vi "烧录座位置补偿设定界面.vi"(8 "错误输入（无错误）":errorcluster, 10 "界面切换队列":refnum<queue>, 11 "VISA资源名称输入":refnum<visa-resource-name>) -> (0 "错误输出":errorcluster, 3 "VISA资源名称输出":refnum<visa-resource-name>)   [LabVIEW 2018]
panel:
  out "毫秒计时值":u32
  in  "枚举":T1(ring)
  in  "选项卡控件":enum32{"选项卡 1", "选项卡 2"}(tab)
  out "吸嘴偏移参数界面":bool
  out "写DDT32480":dbl
  out "写DDT32430":dbl
  out "写DDT32478":dbl
  out "写DDT32428":dbl
  out "写DDT32476":dbl
  out "写DDT32426":dbl
  out "写DDT32474":dbl
  out "写DDT32424":dbl
  out "写DDT32472":dbl
  out "写DDT32422":dbl
  out "写DDT32470":dbl
  out "写DDT32420":dbl
  out "写DDT32468":dbl
  out "写DDT32418":dbl
  out "写DDT32466":dbl
  out "写DDT32416":dbl
  out "写DDT32464":dbl
  out "写DDT32414":dbl
  out "写DDT32462":dbl
  out "写DDT32412":dbl
  out "写DDT32460":dbl
  out "写DDT32410":dbl
  out "写DDT32458":dbl
  out "写DDT32408":dbl
  out "写DDT32456":dbl
  out "写DDT32406":dbl
  out "写DDT32454":dbl
  out "写DDT32404":dbl
  out "写DDT32452":dbl
  out "写DDT32402":dbl
  out "写DDT32450":dbl
  out "写DDT32400":dbl
  out "DDT90356":dbl
  out "DDT90348":dbl
  out "自动界面":bool
  out "手动界面":bool
  out "参数界面":bool
  out "IO界面":bool
  out "产品界面":bool
  out "字符串":string
  out "DDT90352":dbl
  out "DDT90360":dbl
  out "通讯周期":dbl
  out "DT1184":T2(ring)
  out "写R0+读R1+手动启动":bool
  out "写R4+读R4+手动停止":bool
  out "写R8+读R9+机器复位":bool
  # "X"
  # "Z1"
  # "Z2"
  # "Y"
  # "Y轴"
  # "Y轴"
  # "X轴"
  # "X轴"
  # "烧录座补偿"
  # "09"
  # "01"
  # "只有光标\n对位模式下\n补偿才有用"
  # "10"
  # "02"
  # "11"
  # "03"
  # "要多走一点\n就设正值\n要少走一点\n就设负值\n比如要多走1MM\n就设1.00\n如果想要少走1MM\n就设-1.00"
  # "12"
  # "04"
  # "13"
  # "05"
  # "14"
  # "06"
  # "15"
  # "07"
  # "16"
  # "08"
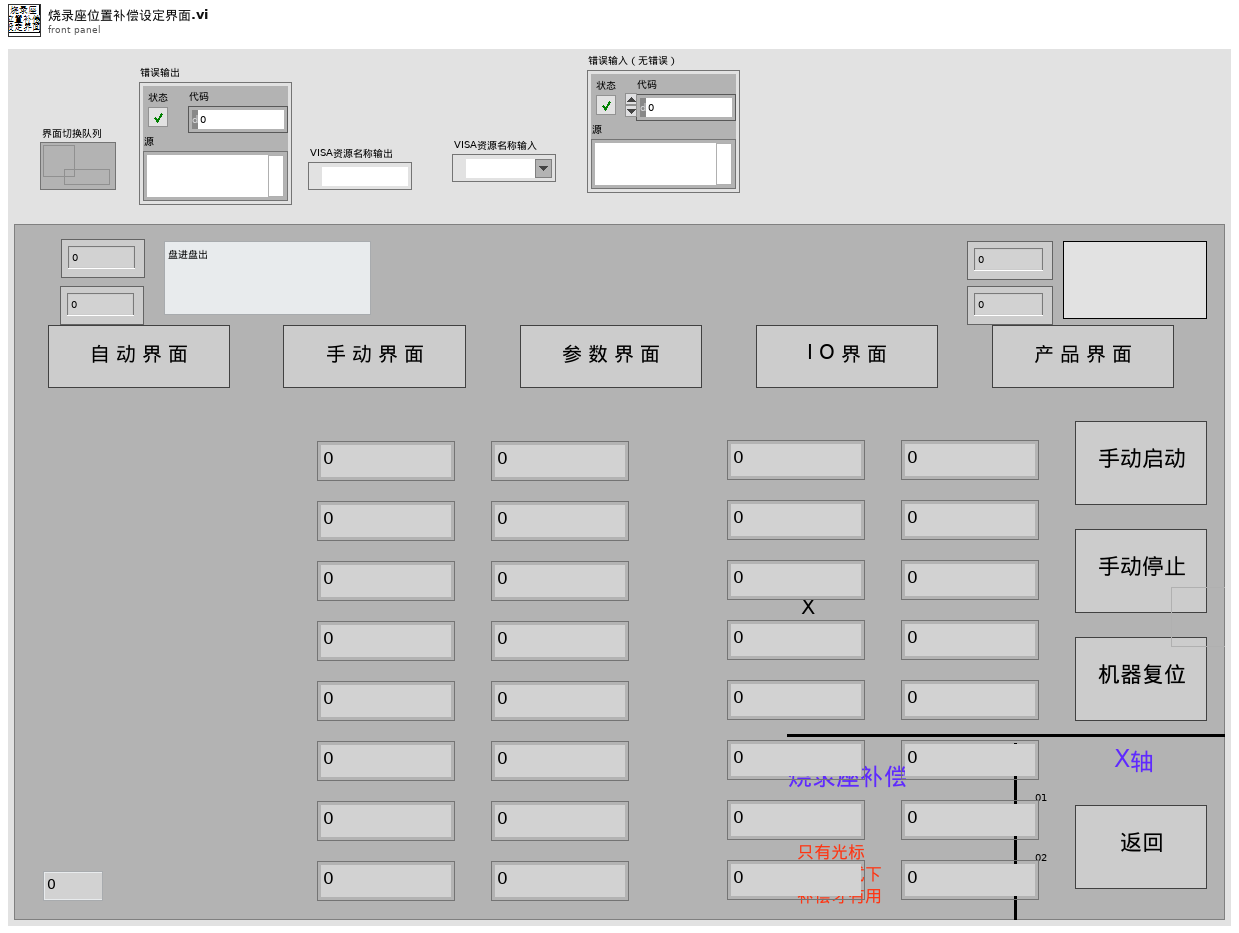
[diagram p1: front panel]
types:
  T1 = enum16{"读初始化", "读R9+8", "读R1+8", "读DDT32480", "读DDT32470+5", "读DDT32460+5", "读DDT32450+5", "读DDT32430", "读DDT32420+5", "读DDT32410+5", "读DDT32400+5", "读DDT90356", "读DT1184", "读DDT90348", ""}
  T2 = enum16{"盘进盘出", "卷进卷出", "盘进卷出", "管进盘出", "管进卷出", "卷进盘出", ""}
  T3 = enum8{"Enabled", "Disabled", "Disabled and Grayed Out"}
  T4 = typedef "数据簇.ctl" = cluster{"字符串":string, "数值":i32, "布尔":bool}
  T5 = typedef "lveventtype.ctl" = enum32{"Null", "Timeout", "Annotation Menu Selection", "Annotation Menu Selection?", "App Instance Close", "App Instance Close?", "Autoscale Range Change", "Bookmark Info Change", "Cell Edit", "Cell Edit?", "Cursor Grab", "Cursor Grab?", "Cursor Menu Selection", "Cursor Menu Selection?", "Cursor Move", "Cursor Release", "Data Change", "Direction Change", "Display State Change", "Drag Ended", "Drag Enter", "Drag Leave", "Drag Over", "Drag Source Update", "Drag Starting", "Drag Starting?", "Drop", "Exec State Change", "Key Down", "Key Down?", "Key Repeat", "Key Repeat?", "Key Up", "Listbox Double Click", "Menu Activation?", "Menu Selection (App)", "Menu Selection? (App)", "Menu Selection (User)", "Mouse Down", "Mouse Down?", "Mouse Enter", "Mouse Leave", "Mouse Move", "Mouse Up", "Mouse Wheel", "NI Security User Change (App)", "Pane Size", "Panel Close", "Panel Close?", "Panel Resize", "Plot Attribute Change", "Scale Range Change", "Shortcut Menu Activation?", "Shortcut Menu Selection (App)", "Shortcut Menu Selection? (App)", "Shortcut Menu Selection (User)", "Tree Double Click", "Tree Drag", "Tree Drag?", "Tree Drop", "Tree Drop?", "Tree Item Close", "Tree Item Close?", "Tree Item Open", "Tree Item Open?", "User Event", "Value Change"}
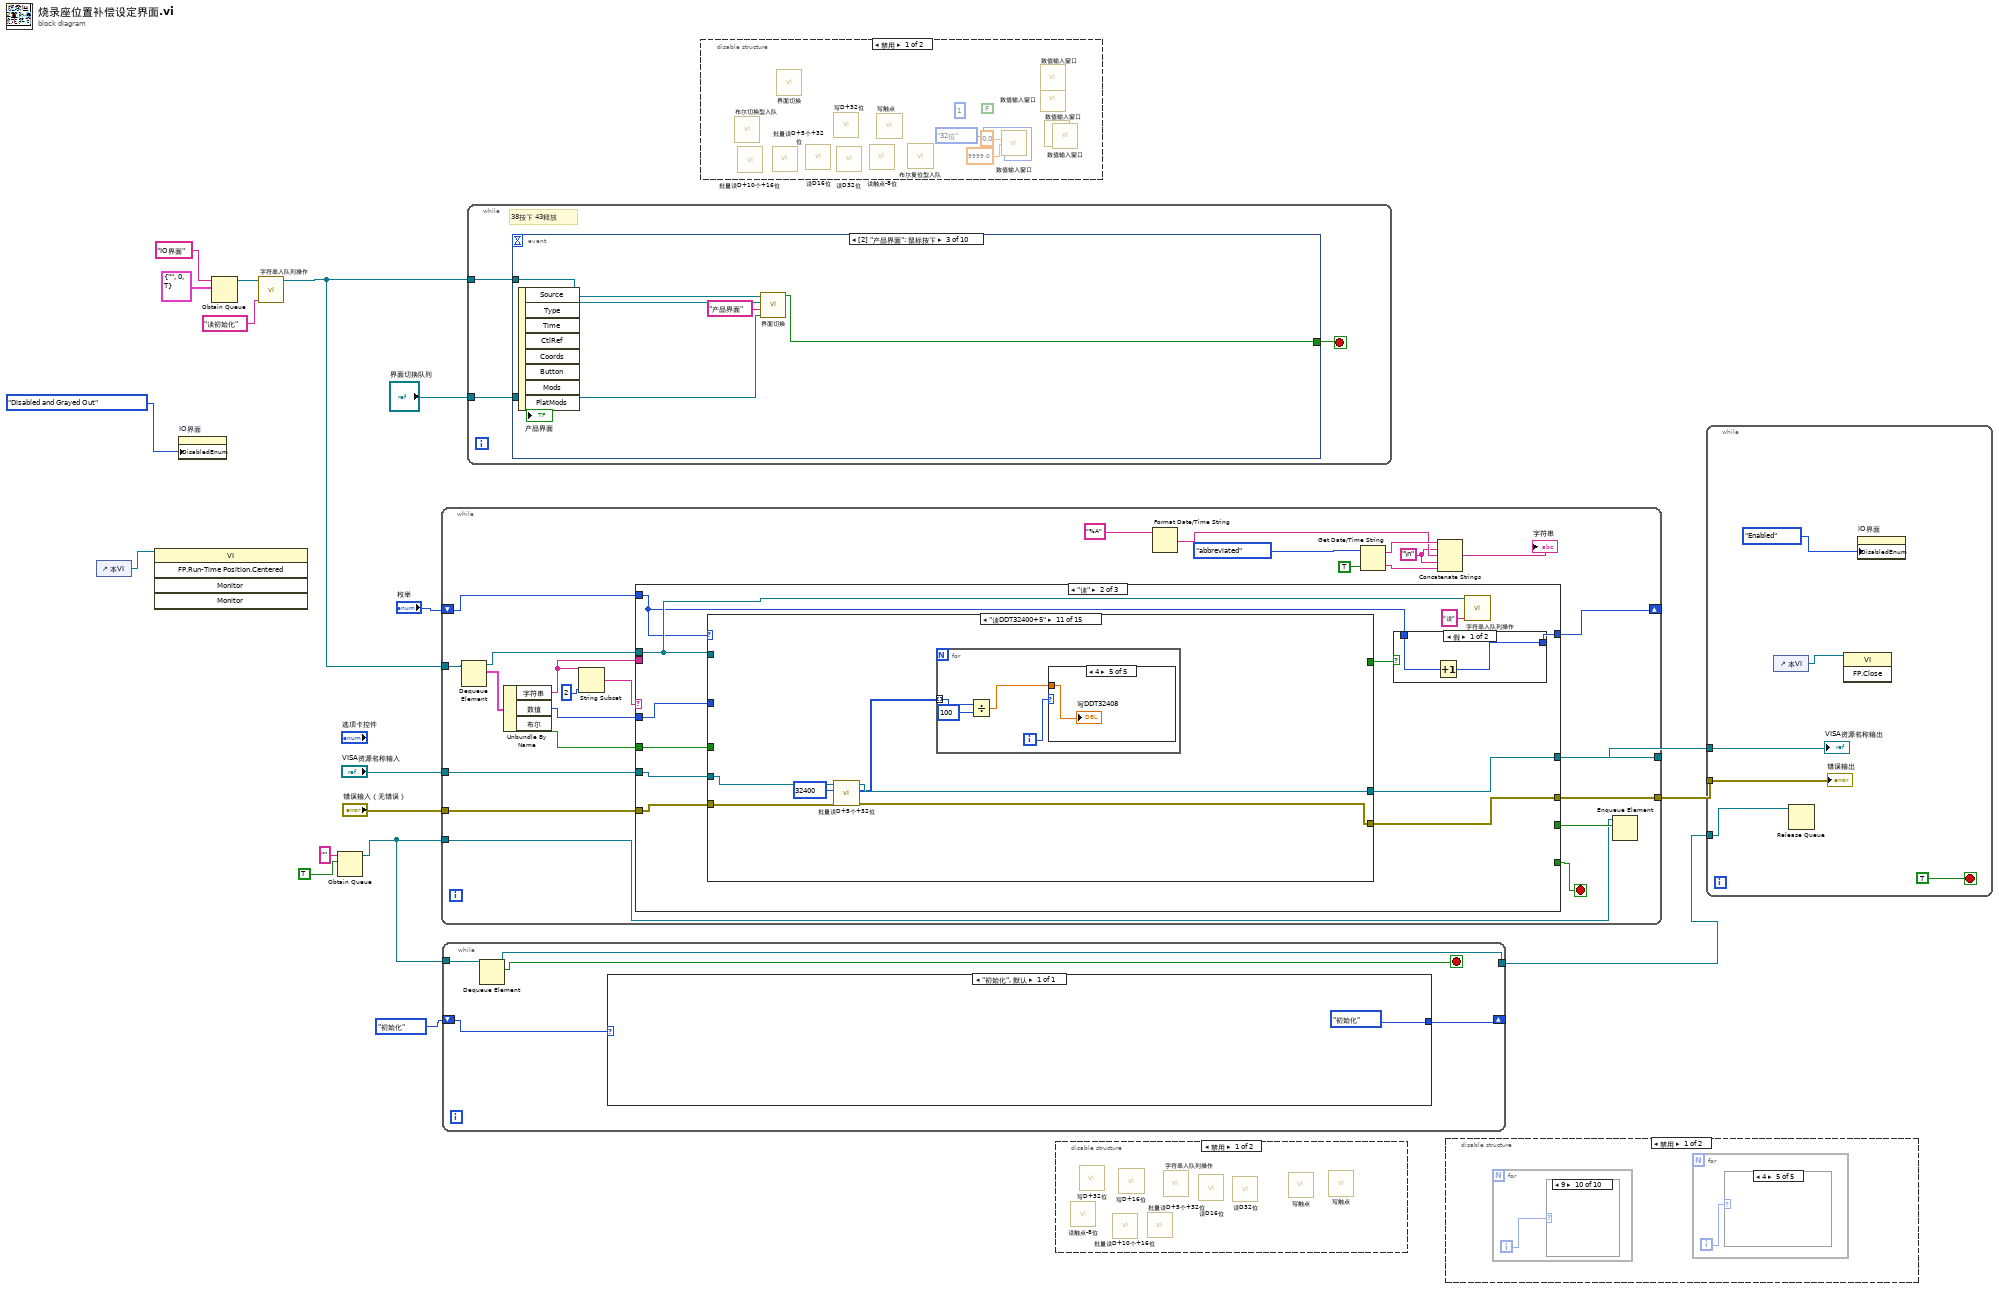
[diagram p0: block diagram]
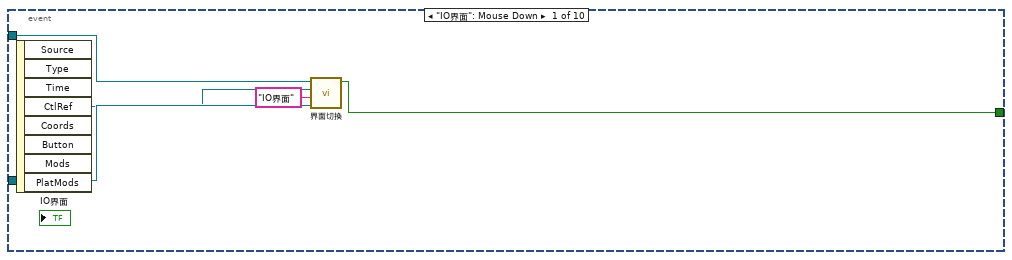
[diagram p18: hidden frame]
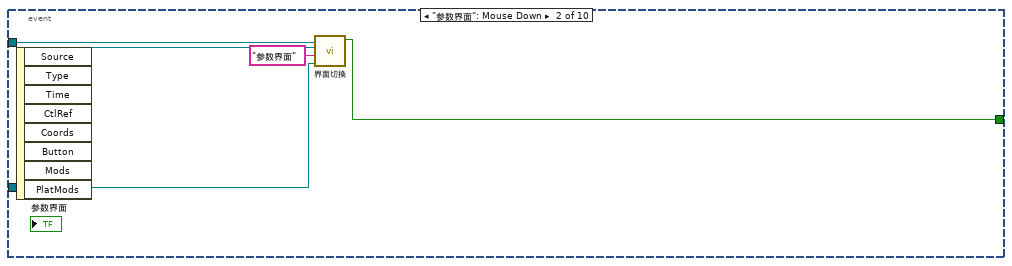
[diagram p19: hidden frame]
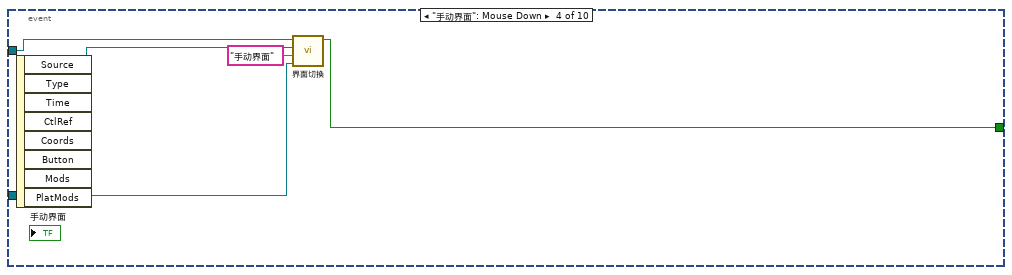
[diagram p20: hidden frame]
diagram:
  n1 = control-ref of="本VI"() -> (w1:refnum<vi>)
  n2 = invoke class="VI" method="FP.Run-Time Position.Centered"(reference=w1) -> ()  [unwired: 4 in, 5 out]
  n3 = property on="IO界面" class="Bool"("DisabledEnum"=T3."Disabled and Grayed Out" ("禁用")) -> ()  [unwired: 2 in, 2 out]
  n4 = Obtain Queue(name (unnamed)="IO界面" ("名称（未命名）"), element data type=T4 {"字符串"="", "数值"=0, "布尔"=TRUE}) -> (queue out=w11:refnum<queue>)  [unwired: 3 in, 2 out]
  n5 = call "字符串入队列操作.vi"("字符消息入队列"="读初始化", "界面切换队列"=w11) -> ("队列输出"=w3:refnum<queue>)  [unwired: 9 in]
  n6 = Obtain Queue(name (unnamed)="" ("名称（未命名）"), element data type=TRUE) -> (queue out=w6:refnum<queue>)  [unwired: 3 in, 2 out]
  n7 = while {
    tunnel: w3 -> [w39]
    tunnel: "VISA资源名称输入" -> [w32]
    tunnel: "错误输入（无错误）" -> [w31]
    tunnel: [w30] -> w13
    tunnel: [w29] -> w12
    shift-right: [w26] -> _
    shift-left: "枚举" -> [w27]
    tunnel: w6 -> [w19]
    stop <- w21 stop-if-true
    w23 = "\n"
    n8 = Dequeue Element(queue=w39) -> (queue out=w36:refnum<queue>, element=w38:T4)  [unwired: 2 in, 2 out]
    n9 = Unbundle By Name(w38) -> ("字符串"=w33:string, "数值"=w35:i32, "布尔"=w34:bool)
    n10 = String Subset(string=w33, length (rest)=2 ("长度（剩余）")) -> (substring=w37:string)  [unwired: 1 in]
    n11 = case shown="\"读\"" w37 {
      selector: w37 -> [w46 _ _]
      tunnel: w36 -> [_ w54 w250]
      tunnel: w35 -> [_ w61 w249]
      tunnel: w34 -> [_ w60 w248]
      tunnel: w33 -> [_ _ w242]
      tunnel: w32 -> [w45 w59 w247]
      tunnel: w31 -> [w44 w58 w246]
      tunnel: [w45 w57 w244] -> w30
      tunnel: [w44 w56 w243] -> w29
      tunnel: [_ _ w245] -> w21
      tunnel: w27 -> [_ w52 _]
      tunnel: [_ w51 _] -> w26
      tunnel: [_ _ w240] -> w20
      frame "", Default {
        n12 = Concatenate Strings("无对应消息分支**" ("消息"), w46, "**" ("字符串"), "读写状态机" ("字符串")) -> (w48:string)
        n13 = One Button Dialog(message=w48) -> ()  [unwired: 1 in, 1 out]
      }
      frame "读" {
        n14 = case shown="\"读DDT32400+5\"" w52 {
          tunnel: w54 -> [_ _ _ _ _ _ _ _ _ _ _ _ _ _ _]
          tunnel: w61 -> [_ _ _ _ _ _ _ _ _ _ _ _ _ _ _]
          tunnel: w59 -> [w66 w73 w83 w95 w101 w116 w131 w148 w154 w169 w184 w205 w214 w227 w239]
          tunnel: w58 -> [w65 w72 w82 w94 w100 w115 w130 w147 w153 w168 w183 w204 w213 w226 w238]
          tunnel: [w66 w69 w79 w92 w98 w113 w128 w145 w151 w166 w182 w203 w212 w225 w239] -> w57
          tunnel: [w65 w68 w78 w91 w97 w112 w127 w144 w150 w165 w181 w202 w211 w224 w238] -> w56
          tunnel: w60 -> [_ _ _ _ _ _ _ _ _ _ _ _ _ _ _]
          tunnel: [_ _ _ _ _ _ _ _ _ _ _ _ _ _ TRUE] -> w53
          frame "读初始化" {
            n15 = Tick Count (ms)() -> (millisecond timer value=→"毫秒计时值":u32)
          }
          frame "读R9+8" {
            n16 = call "读触点-8位.vi"("error out"=w72, "触点类型"="R", "读取起始地址"="9", "VISA resource name out"=w73) -> ("error IO"=w68:errorcluster, "读取布尔数组"=w67:bool[], "VISA resource name out 2"=w69:refnum<visa-resource-name>)  [unwired: 4 in, 1 out]
            n17 = for {
              tunnel: w67 -> [w74] mode=indexing
              i -> [w75]
              n18 = case shown="0, 默认" w75 {
                tunnel: w74 -> [w76 _ _ _ _ _ _ _]
                frame 0, Default {
                  "写R8+读R9+机器复位" <- w76
                }
                frame 1 {
                }
                frame 2 {
                }
                frame 3 {
                }
                frame 4 {
                }
                frame 5 {
                }
                frame 6 {
                }
                frame 7 {
                }
              }
            }
          }
          frame "读R1+8" {
            n19 = call "读触点-8位.vi"("error out"=w82, "触点类型"="R", "读取起始地址"="1", "VISA resource name out"=w83) -> ("error IO"=w78:errorcluster, "读取布尔数组"=w77:bool[], "VISA resource name out 2"=w79:refnum<visa-resource-name>)  [unwired: 4 in, 1 out]
            n20 = for {
              tunnel: w77 -> [w84] mode=indexing
              i -> [w85]
              n21 = case shown="3" w85 {
                tunnel: w84 -> [w86 _ _ w87 _ _ _ _]
                frame 0, Default {
                  "写R0+读R1+手动启动" <- w86
                }
                frame 1 {
                }
                frame 2 {
                }
                frame 3 {
                  "写R4+读R4+手动停止" <- w87
                }
                frame 4 {
                }
                frame 5 {
                }
                frame 6 {
                }
                frame 7 {
                }
              }
            }
          }
          frame "读DDT32480" {
            n22 = call "读D32位.vi"("error out"=w94, "读取D地址"=32480, "VISA resource name out"=w95) -> ("error IO"=w91:errorcluster, "数值"=w90:i32, "VISA resource name out 2"=w92:refnum<visa-resource-name>)  [unwired: 6 in]
            n23 = Divide(x=w90, y=100) -> (x/y=→"写DDT32480":dbl)
          }
          frame "读DDT32470+5" {
            n24 = call "批量读D+5个+32位.vi"("error out"=w100, "读取D地址"=32470, "VISA resource name out"=w101) -> ("error IO"=w97:errorcluster, "数组"=w96:i32[], "VISA resource name out 2"=w98:refnum<visa-resource-name>)  [unwired: 5 in, 1 out]
            n25 = for {
              tunnel: w96 -> [w104] mode=indexing
              i -> [w105]
              n26 = Divide(x=w104, y=100) -> (x/y=w102:dbl)
              n27 = case shown="4" w105 {
                tunnel: w102 -> [w106 w107 w108 w109 w110]
                frame 0, Default {
                  "写DDT32470" <- w106
                }
                frame 1 {
                  "写DDT32472" <- w107
                }
                frame 2 {
                  "写DDT32474" <- w108
                }
                frame 3 {
                  "写DDT32476" <- w109
                }
                frame 4 {
                  "写DDT32478" <- w110
                }
              }
            }
          }
          frame "读DDT32460+5" {
            n28 = call "批量读D+5个+32位.vi"("error out"=w115, "读取D地址"=32460, "VISA resource name out"=w116) -> ("error IO"=w112:errorcluster, "数组"=w111:i32[], "VISA resource name out 2"=w113:refnum<visa-resource-name>)  [unwired: 5 in, 1 out]
            n29 = for {
              tunnel: w111 -> [w119] mode=indexing
              i -> [w120]
              n30 = Divide(x=w119, y=100) -> (x/y=w117:dbl)
              n31 = case shown="4" w120 {
                tunnel: w117 -> [w121 w122 w123 w124 w125]
                frame 0, Default {
                  "写DDT32460" <- w121
                }
                frame 1 {
                  "写DDT32462" <- w122
                }
                frame 2 {
                  "写DDT32464" <- w123
                }
                frame 3 {
                  "写DDT32466" <- w124
                }
                frame 4 {
                  "写DDT32468" <- w125
                }
              }
            }
          }
          frame "读DDT32450+5" {
            n32 = call "批量读D+5个+32位.vi"("error out"=w130, "读取D地址"=32450, "VISA resource name out"=w131) -> ("error IO"=w127:errorcluster, "数组"=w126:i32[], "VISA resource name out 2"=w128:refnum<visa-resource-name>)  [unwired: 5 in, 1 out]
            n33 = for {
              tunnel: w126 -> [w134] mode=indexing
              i -> [w135]
              n34 = Divide(x=w134, y=100) -> (x/y=w132:dbl)
              n35 = case shown="4" w135 {
                tunnel: w132 -> [w136 w137 w138 w139 w140]
                frame 0, Default {
                  "写DDT32450" <- w136
                }
                frame 1 {
                  "写DDT32452" <- w137
                }
                frame 2 {
                  "写DDT32454" <- w138
                }
                frame 3 {
                  "写DDT32456" <- w139
                }
                frame 4 {
                  "写DDT32458" <- w140
                }
              }
            }
          }
          frame "读DDT32430" {
            n36 = call "读D32位.vi"("error out"=w147, "读取D地址"=32430, "VISA resource name out"=w148) -> ("error IO"=w144:errorcluster, "数值"=w143:i32, "VISA resource name out 2"=w145:refnum<visa-resource-name>)  [unwired: 6 in]
            n37 = Divide(x=w143, y=100) -> (x/y=→"写DDT32430":dbl)
          }
          frame "读DDT32420+5" {
            n38 = call "批量读D+5个+32位.vi"("error out"=w153, "读取D地址"=32420, "VISA resource name out"=w154) -> ("error IO"=w150:errorcluster, "数组"=w149:i32[], "VISA resource name out 2"=w151:refnum<visa-resource-name>)  [unwired: 5 in, 1 out]
            n39 = for {
              tunnel: w149 -> [w157] mode=indexing
              i -> [w158]
              n40 = Divide(x=w157, y=100) -> (x/y=w155:dbl)
              n41 = case shown="4" w158 {
                tunnel: w155 -> [w159 w160 w161 w162 w163]
                frame 0, Default {
                  "写DDT32420" <- w159
                }
                frame 1 {
                  "写DDT32422" <- w160
                }
                frame 2 {
                  "写DDT32424" <- w161
                }
                frame 3 {
                  "写DDT32426" <- w162
                }
                frame 4 {
                  "写DDT32428" <- w163
                }
              }
            }
          }
          frame "读DDT32410+5" {
            n42 = call "批量读D+5个+32位.vi"("error out"=w168, "读取D地址"=32410, "VISA resource name out"=w169) -> ("error IO"=w165:errorcluster, "数组"=w164:i32[], "VISA resource name out 2"=w166:refnum<visa-resource-name>)  [unwired: 5 in, 1 out]
            n43 = for {
              tunnel: w164 -> [w172] mode=indexing
              i -> [w173]
              n44 = Divide(x=w172, y=100) -> (x/y=w170:dbl)
              n45 = case shown="4" w173 {
                tunnel: w170 -> [w174 w175 w176 w177 w178]
                frame 0, Default {
                  "写DDT32410" <- w174
                }
                frame 1 {
                  "写DDT32412" <- w175
                }
                frame 2 {
                  "写DDT32414" <- w176
                }
                frame 3 {
                  "写DDT32416" <- w177
                }
                frame 4 {
                  "写DDT32418" <- w178
                }
              }
            }
          }
          frame "读DDT32400+5" {
            n46 = call "批量读D+5个+32位.vi"("error out"=w183, "读取D地址"=32400, "VISA resource name out"=w184) -> ("error IO"=w181:errorcluster, "数组"=w179:i32[], "VISA resource name out 2"=w182:refnum<visa-resource-name>)  [unwired: 5 in, 1 out]
            n47 = for {
              tunnel: w179 -> [w187] mode=indexing
              i -> [w188]
              n48 = Divide(x=w187, y=100) -> (x/y=w185:dbl)
              n49 = case shown="4" w188 {
                tunnel: w185 -> [w189 w190 w191 w192 w193]
                frame 0, Default {
                  "写DDT32400" <- w189
                }
                frame 1 {
                  "写DDT32402" <- w190
                }
                frame 2 {
                  "写DDT32404" <- w191
                }
                frame 3 {
                  "写DDT32406" <- w192
                }
                frame 4 {
                  "写DDT32408" <- w193
                }
              }
            }
          }
          frame "读DDT90356" {
            n50 = call "批量读D+5个+32位.vi"("error out"=w204, "读取D地址"=90356, "VISA resource name out"=w205) -> ("error IO"=w202:errorcluster, "数组"=w208:i32[], "VISA resource name out 2"=w203:refnum<visa-resource-name>)  [unwired: 5 in, 1 out]
            n51 = Index Array(array=w208, index #1=0 ("索引"), index #2=2 ("索引")) -> (element #1=w201:i32, element #2=w200:i32)
            n52 = To Double Precision Float(number=w201) -> (double precision float=w199:dbl)
            n53 = To Double Precision Float(number=w200) -> (double precision float=w196:dbl)
            n54 = Divide(x=w199, y=100.0) -> (x/y=→"DDT90356":dbl)
            n55 = Divide(x=w196, y=100.0) -> (x/y=→"DDT90360":dbl)
          }
          frame "读DT1184" {
            n56 = call "读D16位.vi"("error out"=w213, "读取D地址"=1184, "VISA resource name out"=w214) -> ("error IO"=w211:errorcluster, "数值"=→"DT1184":u32, "VISA resource name out 2"=w212:refnum<visa-resource-name>)  [unwired: 5 in, 1 out]
          }
          frame "读DDT90348" {
            n57 = call "批量读D+5个+32位.vi"("error out"=w226, "读取D地址"=90348, "VISA resource name out"=w227) -> ("error IO"=w224:errorcluster, "数组"=w231:i32[], "VISA resource name out 2"=w225:refnum<visa-resource-name>)  [unwired: 5 in, 1 out]
            n58 = Index Array(array=w231, index #1=0 ("索引"), index #2=2 ("索引")) -> (element #1=w223:i32, element #2=w222:i32)
            n59 = To Double Precision Float(number=w222) -> (double precision float=w217:dbl)
            n60 = To Double Precision Float(number=w223) -> (double precision float=w221:dbl)
            n61 = Divide(x=w217, y=100.0) -> (x/y=→"DDT90352":dbl)
            n62 = Divide(x=w221, y=100.0) -> (x/y=→"DDT90348":dbl)
          }
          frame "" {
            n63 = local read "毫秒计时值"() -> (w235:u32)
            n64 = Tick Count (ms)() -> (millisecond timer value=w236:u32)
            n65 = Subtract(x=w236, y=w235) -> (x-y=w234:u32)
            n66 = Divide(x=w234, y=u32 1000) -> (x/y=→"通讯周期":dbl)
          }
        }
        n67 = case shown="假" w53 {
          tunnel: w52 -> [w63 _]
          tunnel: [w62 _] -> w51
          frame False {
            n68 = Increment(x=w63) -> (x+1=w62:T1)
          }
          frame True {
          }
        }
        n69 = call "字符串入队列操作.vi"("字符消息入队列"="读", "界面切换队列"=w54) -> ()  [unwired: 9 in, 1 out]
      }
      frame "写" {
        n70 = call "状态匹配.vi"("输入状态"=w242) -> ("输出状态"=w241:string)  [unwired: 10 in]
        n71 = case shown="\"写退出\"" w241 {
          selector: w241 -> [w253 _ _ _ _]
          tunnel: w250 -> [_ _ _ _ w293]
          tunnel: w249 -> [_ w259 w276 _ _]
          tunnel: w248 -> [_ _ _ w287 _]
          tunnel: w247 -> [w252 w269 w280 w292 w298]
          tunnel: w246 -> [w251 w268 w279 w291 w297]
          tunnel: [_ _ _ _ w296] -> w245
          tunnel: [w252 w267 w278 w290 w298] -> w244
          tunnel: [w251 w266 w277 w289 w297] -> w243
          tunnel: w242 -> [_ w258 w270 w281 _]
          tunnel: [_ _ _ _ w296] -> w240
          frame "", Default {
            n72 = Concatenate Strings("无对应消息分支**" ("消息"), w253, "**" ("字符串"), "写状态机" ("字符串")) -> (w257:string)
            n73 = One Button Dialog(message=w257) -> ()  [unwired: 1 in, 1 out]
          }
          frame "写DT" {
            n74 = String Length(string=w258) -> (length=w264:i32)
            n75 = Subtract(x=w264, y=4) -> (x-y=w262:i32)
            n76 = String Subset(string=w258, offset (0)=4 ("偏移量(0)"), length (rest)=w262) -> (substring=w261:string)
            n77 = Decimal String To Number(string=w261) -> (number=w260:i32)  [unwired: 2 in, 1 out]
            n78 = call "写D+16位.vi"("error out"=w268, "输入数值"=w259, "输入地址D"=w260, "VISA resource name out"=w269) -> ("error out 2"=w266:errorcluster, "VISA resource name out 2"=w267:refnum<visa-resource-name>)  [unwired: 3 in, 3 out]
          }
          frame "写DDT" {
            n79 = String Length(string=w270) -> (length=w274:i32)
            n80 = Subtract(x=w274, y=5) -> ()  [unwired: 1 out]
            n81 = String Subset(string=w270, offset (0)=5 ("偏移量(0)")) -> (substring=w271:string)  [unwired: 1 in]
            n82 = Decimal String To Number(string=w271) -> (number=w272:i32)  [unwired: 2 in, 1 out]
            n83 = call "写D+32位.vi"("error out"=w279, "输入数值"=w276, "输入地址D"=w272, "VISA resource name out"=w280) -> ("error out 2"=w277:errorcluster, "VISA resource name out 2"=w278:refnum<visa-resource-name>)  [unwired: 4 in, 2 out]
          }
          frame "写R" {
            n84 = String Length(string=w281) -> (length=w285:i32)
            n85 = Subtract(x=w285, y=3) -> (x-y=w283:i32)
            n86 = String Subset(string=w281, offset (0)=3 ("偏移量(0)"), length (rest)=w283) -> (substring=w282:string)
            n87 = call "写触点.vi"("布尔"=w287, "error out"=w291, "触点类型"="R", "写入起始地址"=w282, "VISA resource name out"=w292) -> ("error IO"=w289:errorcluster, "VISA resource name out 2"=w290:refnum<visa-resource-name>)  [unwired: 4 in, 1 out]
          }
          frame "写退出" {
            w296 = TRUE
            n88 = Flush Queue(queue=w293) -> (queue out=w294:refnum<queue>, error out=w295:errorcluster)  [unwired: 1 in, 1 out]
            n89 = Release Queue(queue=w294, error in (no error)=w295) -> ()  [unwired: 1 in, 3 out]
          }
        }
      }
    }
    n90 = Format Date/Time String(time format string (%c)="%A" ("时间格式字符串(%c)")) -> (date/time string=w24:string)  [unwired: 2 in]
    n91 = Get Date/Time String(date format (0)=enum16{"short", "long", "abbreviated"}."abbreviated" ("日期格式(0)"), want seconds? (F)=TRUE ("需要秒？(F)")) -> (date string=w41:string, time string=w22:string)  [unwired: 1 in]
    n92 = Concatenate Strings(w41, w23, w24, w23, w22) -> (→"字符串":string)
    n93 = Enqueue Element(queue=w19, element=w20) -> ()  [unwired: 2 in, 3 out]
  }
  n94 = while {
    shift-right: [w302] -> _
    shift-left: enum16{"初始化"}."初始化" -> [w303]
    tunnel: w6 -> [w301]
    tunnel: [w299] -> w5
    stop <- w300 stop-if-true
    n95 = Dequeue Element(queue=w301) -> (queue out=w299:refnum<queue>, element=w300:bool)  [unwired: 2 in, 2 out]
    n96 = case shown="\"初始化\", 默认" w303 {
      tunnel: [enum16{"初始化"}."初始化"] -> w302
      frame "初始化", Default {
      }
    }
  }
  n97 = while {
    tunnel: w3 -> [w306]
    tunnel: "界面切换队列" -> [w305]
    stop <- w307 stop-if-true
    # "38按下 43释放"
    n98 = event shown="[2] \"产品界面\": 鼠标按下" {
      selector: _ -> [_ _ _ _ _ _ _ _ _ _]
      dyn-events: _ -> [_ _ _ _ _ _ _ _ _ _]
      timeout: _ -> [_ _ _ _ _ _ _ _ _ _]
      tunnel: [w311 w313 w318 w323 w328 _ _ w348 _ w355] -> w307
      tunnel: w306 -> [w312 w317 w322 w327 w332 w340 w347 w352 _ w354]
      tunnel: w305 -> [w310 w316 w321 w326 w331 _ _ w351 _ w353]
      event "IO界面": Mouse Down {
        n99 = event-data() -> ("CtlRef"=w309:refnum<vi>)  [unwired: 1 in, 7 out]
        n100 = call "界面切换.vi"("界面切换队列输入"=w310, "切换界面名称输入"="IO界面", "Bool引用句柄"=w309, "状态转移输入"=w312) -> ("布尔"=w311:bool)  [unwired: 7 in]
      }
      event "参数界面": Mouse Down {
        n101 = event-data() -> ("CtlRef"=w315:refnum<vi>)  [unwired: 1 in, 7 out]
        n102 = call "界面切换.vi"("界面切换队列输入"=w316, "切换界面名称输入"="参数界面", "Bool引用句柄"=w315, "状态转移输入"=w317) -> ("布尔"=w313:bool)  [unwired: 7 in]
      }
      event "产品界面": Mouse Down {
        n103 = event-data() -> ("CtlRef"=w320:refnum<vi>)  [unwired: 1 in, 7 out]
        n104 = call "界面切换.vi"("界面切换队列输入"=w321, "切换界面名称输入"="产品界面", "Bool引用句柄"=w320, "状态转移输入"=w322) -> ("布尔"=w318:bool)  [unwired: 7 in]
      }
      event "手动界面": Mouse Down {
        n105 = event-data() -> ("CtlRef"=w325:refnum<vi>)  [unwired: 1 in, 7 out]
        n106 = call "界面切换.vi"("界面切换队列输入"=w326, "切换界面名称输入"="手动界面", "Bool引用句柄"=w325, "状态转移输入"=w327) -> ("布尔"=w323:bool)  [unwired: 7 in]
      }
      event "吸嘴偏移参数界面": Value Change {
        n107 = event-data() -> ("CtlRef"=w330:refnum<vi>)  [unwired: 1 in, 5 out]
        n108 = call "界面切换.vi"("界面切换队列输入"=w331, "切换界面名称输入"="吸嘴偏移参数界面", "Bool引用句柄"=w330, "状态转移输入"=w332) -> ("布尔"=w328:bool)  [unwired: 7 in]
      }
      event "写DDT32456", "写DDT32402", "写DDT32450", "写DDT32452", "写DDT32404", "写DDT32454", "写DDT32406", "写DDT32458", "写DDT32408", "写DDT32410", "写DDT32460", "写DDT32412", "写DDT32462", "写DDT32414", "写DDT32464", "写DDT32416", "写DDT32466", "写DDT32418", "写DDT32468", "写DDT32420", "写DDT32470", "写DDT32422", "写DDT32472", "写DDT32424", "写DDT32474", "写DDT32426", "写DDT32476", "写DDT32428", "写DDT32478", "写DDT32430", "写DDT32480": Mouse Down {
        n109 = event-data() -> ("CtlRef"=w339:refnum<vi>)  [unwired: 1 in, 7 out]
        n110 = property class="DigNum (严格)"(reference=w339) -> (reference out=w337:refnum<vi>, "Label.Text"=w338:string)  [unwired: 1 in, 1 out]
        n111 = call "数值输入窗口.vi"("消息入队"=w340, "字符串"=w338, "字符消息入队列"=w338, "输入下限"=-99999999.0, "输入上限"=99999999.0, "转换比例"=u32 100, "数据类型"=enum16{"32位", "16位"}."32位", "控件引用"=w337) -> ()  [unwired: 5 in, 3 out]
      }
      event "写R8+读R9+机器复位", "写R4+读R4+手动停止", "写R0+读R1+手动启动": Mouse Down; "写R8+读R9+机器复位", "写R4+读R4+手动停止", "写R0+读R1+手动启动": Mouse Up {
        n112 = event-data() -> ("Type"=w346:T5, "CtlRef"=w345:refnum<vi>)  [unwired: 1 in, 6 out]
        n113 = property class="Bool"(reference=w345) -> (reference out=w344:refnum<vi>, "Label.Text"=w343:string)  [unwired: 1 in, 1 out]
        n114 = Match Pattern(string=w343, regular expression="+" ("正则表达式")) -> (before substring=w341:string)  [unwired: 1 in, 3 out]
        n115 = call "布尔复位型入队.vi"("队列输入"=w347, "数值"=w346, "控件引用"=w344, "字符消息入队列"=w341) -> ()  [unwired: 2 in, 3 out]
      }
      event "自动界面": Mouse Down {
        n116 = event-data() -> ("CtlRef"=w350:refnum<vi>)  [unwired: 1 in, 7 out]
        n117 = call "界面切换.vi"("界面切换队列输入"=w351, "切换界面名称输入"="自动界面", "Bool引用句柄"=w350, "状态转移输入"=w352) -> ("布尔"=w348:bool)  [unwired: 7 in]
      }
      event Timeout {
        n118 = event-data() -> ()  [unwired: 1 in, 3 out]
      }
      event Panel Close? {
        n119 = event-data() -> ()  [unwired: 1 in, 4 out]
        n120 = Two Button Dialog(message="确定退出程序？" ("消息")) -> (T button?=w356:bool)  [unwired: 2 in]
        n121 = case shown="真" w356 {
          tunnel: [_ TRUE] -> w355
          tunnel: w354 -> [_ w361]
          tunnel: w353 -> [_ w360]
          frame False {
          }
          frame True {
            n122 = call "字符串入队列操作.vi"("字符消息入队列"="退出", "界面切换队列"=w360) -> ()  [unwired: 9 in, 1 out]
            n123 = call "字符串入队列操作.vi"("字符消息入队列"="写退出", "界面切换队列"=w361) -> ()  [unwired: 9 in, 1 out]
          }
        }
        n124 = event-data("Discard?"=TRUE ("放弃？")) -> ()  [unwired: 1 in, 1 out]
      }
    }
  }
  n125 = disable-structure shown="禁用" {
    frame Disabled {
      (unwired) u32 1 ("转换比例")
      (unwired) FALSE ("忽略数值上下限")
      n126 = call "布尔切换型入队.vi"() -> ()  [unwired: 12 in]
      n127 = call "批量读D+10个+16位.vi"() -> ()  [unwired: 8 in, 4 out]
      n128 = call "批量读D+5个+32位.vi"() -> ()  [unwired: 8 in, 4 out]
      n129 = call "界面切换.vi"() -> ()  [unwired: 11 in, 1 out]
      n130 = call "读D16位.vi"() -> ()  [unwired: 8 in, 4 out]
      n131 = call "写D+32位.vi"() -> ()  [unwired: 8 in, 4 out]
      n132 = call "读D32位.vi"() -> ()  [unwired: 9 in, 3 out]
      n133 = call "读触点-8位.vi"() -> ()  [unwired: 8 in, 4 out]
      n134 = call "写触点.vi"() -> ()  [unwired: 9 in, 3 out]
      n135 = call "布尔复位型入队.vi"() -> ()  [unwired: 6 in, 3 out]
      n136 = call "数值输入窗口.vi"("输入下限"=0.0, "输入上限"=9999.0, "数据类型"=enum16{"32位", "16位"}."32位") -> ("转换比例"=w367:u32)  [unwired: 9 in, 3 out]
      n137 = call "数值输入窗口.vi"() -> ()  [unwired: 13 in, 3 out]
      n138 = call "数值输入窗口.vi"() -> ()  [unwired: 13 in, 3 out]
      n139 = call "数值输入窗口.vi"() -> ()  [unwired: 13 in, 3 out]
      n140 = call "数值输入窗口.vi"() -> ()  [unwired: 13 in, 3 out]
    }
    frame Enabled {
    }
  }
  n141 = disable-structure shown="禁用" {
    frame Disabled {
      n142 = call "读触点-8位.vi"() -> ()  [unwired: 8 in, 4 out]
      n143 = call "写D+32位.vi"() -> ()  [unwired: 8 in, 4 out]
      n144 = call "批量读D+10个+16位.vi"() -> ()  [unwired: 8 in, 4 out]
      n145 = call "写D+16位.vi"() -> ()  [unwired: 7 in, 5 out]
      n146 = call "批量读D+5个+32位.vi"() -> ()  [unwired: 8 in, 4 out]
      n147 = call "字符串入队列操作.vi"() -> ()  [unwired: 11 in, 1 out]
      n148 = call "读D16位.vi"() -> ()  [unwired: 8 in, 4 out]
      n149 = call "读D32位.vi"() -> ()  [unwired: 9 in, 3 out]
      n150 = call "写触点.vi"() -> ()  [unwired: 9 in, 3 out]
      n151 = call "写触点.vi"() -> ()  [unwired: 9 in, 3 out]
    }
    frame Enabled {
    }
  }
  n152 = disable-structure shown="禁用" {
    frame Disabled {
      n153 = for {
        i -> [w369]
        n154 = case shown="9" w369 {
          frame 0, Default {
          }
          frame 1 {
          }
          frame 2 {
          }
          frame 3 {
          }
          frame 4 {
          }
          frame 5 {
          }
          frame 6 {
          }
          frame 7 {
          }
          frame 8 {
          }
          frame 9 {
          }
        }
      }
      n155 = for {
        i -> [w368]
        n156 = case shown="4" w368 {
          frame 0, Default {
          }
          frame 1 {
          }
          frame 2 {
          }
          frame 3 {
          }
          frame 4 {
          }
        }
      }
    }
    frame Enabled {
    }
  }
  n157 = while {
    tunnel: w13 -> [w373]
    tunnel: w12 -> [w372]
    tunnel: w5 -> [w371]
    stop <- TRUE stop-if-true
    n158 = control-ref of="本VI"() -> (w374:refnum<vi>)
    n159 = Release Queue(queue=w371) -> ()  [unwired: 2 in, 3 out]
    n160 = invoke class="VI" method="FP.Close"(reference=w374) -> ()  [unwired: 2 in, 3 out]
    n161 = property on="IO界面" class="Bool"("DisabledEnum"=T3."Enabled" ("禁用")) -> ()  [unwired: 2 in, 2 out]
    "VISA资源名称输出" <- w373
    "错误输出" <- w372
  }
